vi "5785_IQ_gen_2_x_400MHz_max_transfer_back.vi"() -> ()   [LabVIEW 2021]
uses:
  <instrlib>/_niInstr/Streaming/v1/Common/Stream State.ctl
  <vilib>/Platform/TimedLoop/XDataNode/timing_clust.ctl
  <vilib>/Platform/TimedLoop/XDataNode/nitl_modes.ctl
  <vilib>/Platform/TimedLoop/XDataNode/wakeup.ctl
  <instrlib>/FlexRIO/API/FPGA/v1/Types/Start Trigger IO Resources.ctl
  <instrlib>/_niInstr/DSP/v1/Shared/Public/IQ Data.ctl
  <vilib>/rvi/Emulation/niFpgaSctlEmulationGetInTimedLoop.vi
  <vilib>/rvi/Emulation/niFpgaEmulationReportErrorSimple.vi
  <vilib>/rvi/Emulation/niFpgaGetClockAttributes.vi
  <vilib>/rvi/Emulation/niFpgaCriticalErrorInLSC.vi
  <vilib>/rvi/interface/RandomDataEmulation/nirviRandomDataMultiElementFPGAFIFO.vi
  <instcachedir>/0/nirviRandomDataMultiElementFPGAFIFO_3E9965BA1FAD4E7B8DABA31768A09B1F.lvgen/nirviRandomDataMultiElementFPGAFIFO_3E9965BA1FAD4E7B8DABA31768A09B1F_000.vi
  <vilib>/rvi/interface/RandomDataEmulation/niFpgaRandomDataHandleErrors.vi
  7192f61d-e408-4cca-baff-cb10c33219c0.vi
  <instrlib>/_niInstr/DSP/v1/FPGA/Public/Sub VIs/HB Interpolator/Halfband Interpolator - IQ - 2 SPC - 2x OC.vi
  <instrlib>/_niInstr/DSP/v1/FPGA/Public/Sub VIs/Frequency Shift/Frequency Shift - 4 spc.vi
  <instrlib>/_niInstr/DSP/v1/FPGA/Public/Sub VIs/HB Interpolator/Halfband Interpolator - IQ - 4 SPC - 2x OC.vi
  <instrlib>/_niInstr/DSP/v1/FPGA/Public/Sub VIs/HB Interpolator/Halfband Interpolator - IQ - 8 SPC - 2x OC.vi
  <instrlib>/_niInstr/DSP/v1/FPGA/Public/Sub VIs/Frequency Shift/Frequency Shift - 16 spc.vi
  <instrlib>/_niInstr/DSP/v1/FPGA/Public/Sub VIs/HB Decimator/Halfband Decimator - IQ - 16 spc - 2x oc.vi
  <instrlib>/_niInstr/DSP/v1/FPGA/Public/Sub VIs/HB Decimator/Halfband Decimator - IQ - 8 spc - 2x oc.vi
  <instrlib>/_niInstr/DSP/v1/FPGA/Public/Sub VIs/HB Decimator/Halfband Decimator - IQ - 4 spc - 2x oc.vi
  <instrlib>/_niInstr/DSP/v1/FPGA/Public/Sub VIs/Data Conversion/IQ to U32 - 1 spc - S18.1.vi
  <instrlib>/_niInstr/Basic Elements/v1/FPGA/Private/Count Down U32.vi
  <instcachedir>/0/nirviRandomDataMultiElementFPGAFIFO_3E9965BA1FAD4E7B8DABA31768A09B1F.lvgen/nirviRandomDataMultiElementFPGAFIFO_3E9965BA1FAD4E7B8DABA31768A09B1F_003.vi
  <vilib>/rvi/eio/common/nirviEmuTemplateMethod_errors.vi
  <vilib>/Platform/TimedLoop/XDataNode/XDataNode.xnode
  <vilib>/rvi/DataTransferAndStorage/Container/XNode/niFpgaContainer.xnode
  <vilib>/rvi/interface/RandomDataEmulation/nirviRandomDataFpgaMultiElementTemplate.vi
  <vilib>/eio/EIONode/EIONode.xnode
  <vilib>/Platform/TimedLoop/XDataNode/XDNodeRunTimeDep.lvlib
  <instrlib>/_niInstr/Streaming/v1/FPGA/niInstr Streaming v1 FPGA.lvlib
  <instrlib>/FlexRIO/API/FPGA/v1/FlexRIO API FPGA v1.lvlib
  <instrlib>/FlexRIO/API/FPGA/v1/IO/NI5785/FlexRIO 5785 FPGA v1.lvlib
  <instrlib>/_niInstr/DSP/v1/FPGA/niInstr DSP v1 FPGA.lvlib
  <instrlib>/_niInstr/Basic Elements/v1/FPGA/niInstr Basic Elements v1 FPGA.lvlib
  <instrlib>/_niInstr/DSP/v1/Shared/niInstr DSP v1 Shared.lvlib
  <instrlib>/_niInstr/Streaming/v1/Common/niInstr Streaming v1 Common.lvlib
panel:
  out "Is Rx completed":bool
  out "fifo overflow":bool
  in  "rx count .5":u32
  in  "flexrio.stream.channels enabled 1":u64
  in  "frequency shift Tx":fxp<+/-,48,0>
  in  "frequency shift Rx":fxp<+/-,48,0>
  out "pulse TX status 2":T1
  out "pulse TX status":T1
  in  "reset system clock":bool
  in  "User-defined Start Trigger - AO":bool
  in  "flexrio.trigger.start.cfg 1":u16
  out "IO Socket\\AO Ready For Input":bool
  in  "stream.request state 1":T2
  in  "stream.num samples 1":u64
  out "stream.metadata 1":u64
  out "stream.samples transferred 1":u64
  out "stream.state 1":T2
  out "flexrio.module.io ready 0":bool
  out "flexrio.module.io error 0":i32
  out "flexrio.module.data valid 0":bool
  # "Data Path Configuration"
  # "AI Trigger Configuration"
  # "AI Stream Configuration"
  # "AO Stream Configuration"
  # "Module Status"
  # "AO Buffer Configuration"
  # "User-defined Controls"
  # "AO Trigger Configuration"
  # "5785 KU060"
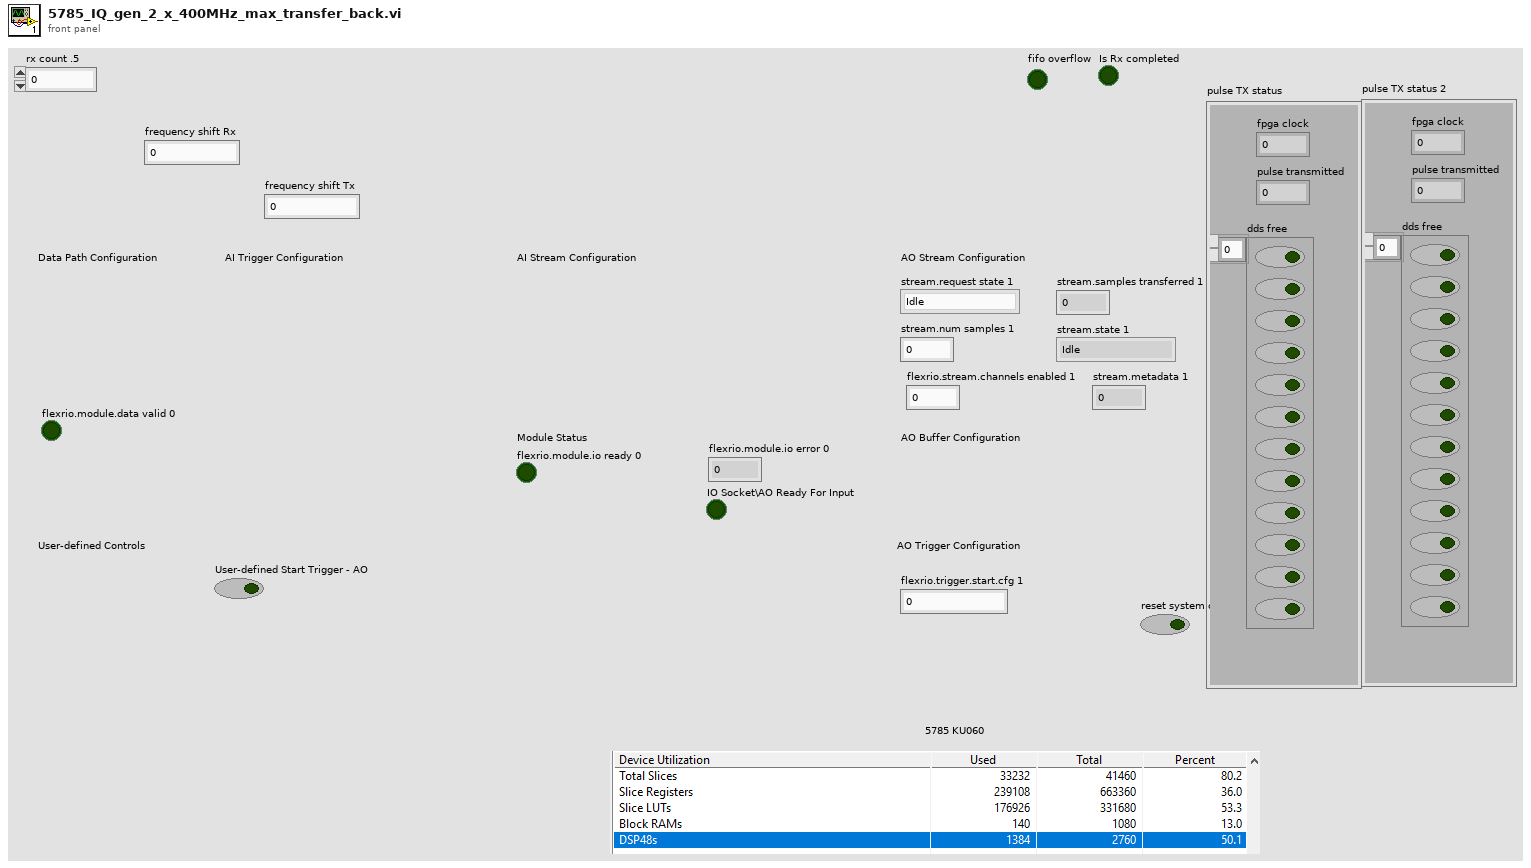
[diagram p1: front panel]
types:
  T1 = cluster{"fpga clock":u64, "pulse transmitted":u32, "dds free":bool[]}
  T2 = typedef "niInstr Streaming v1 Common.lvlib/Stream State.ctl" = enum8{"Idle", "Finite Transfer", "Continuous", "Done", "Error", "Not Ready", "Cancel"}
  T3 = typedef "XDNodeRunTimeDep.lvlib/timing_clust.ctl" = cluster{"Expected End [f-1]":u64, "Actual End [f-1]":u64, "Finished Late? [f-1]":bool, "Expected End [i-1]":u64, "Actual End [i-1]":u64, "Finished Late? [i-1]":bool, "Expected Start [i]":u64, "Actual Start [i]":u64, "Expected Start [f]":u64, "Actual Start [f]":u64, "Source Name":string, "Structure Name":string, "Period":i64, "Deadline":i64, "Offset":i64, "Start":i64, "Priority":i32, "Timeout":i32, "Mode":T4, "Wakeup Reason":T5, "Error":errorcluster, "Source Type":string, "Secondary Source Type":string, "Global End Time":u64, "Global Start Time":u64, "Frame Duration":u64, "Iteration Duration":u64, "Assigned CPU":i32, "I/O Scan Engine Mode":u32}
  T4 = typedef "XDNodeRunTimeDep.lvlib/nitl_modes.ctl" = enum32{"No Change", "Process missed periods, maintain original phase", "Discard missed periods, maintain original phase", "Process missed periods, ignore original phase", "Discard missed periods, ignore original phase"}
  T5 = typedef "XDNodeRunTimeDep.lvlib/wakeup.ctl" = enum32{"Normal", "Aborted", "Asynchronous wakeup", "Timing source error", "Timed loop error", "Timeout"}
  T6 = typedef "FlexRIO API FPGA v1.lvlib/Start Trigger IO Resources.ctl" = cluster{"start trigger":refnum<k21>, "started event":refnum<k21>, "start trigger for export":refnum<k21>, "start trigger for tclk":refnum<k21>}
  T7 = typedef "niInstr DSP v1 Shared.lvlib/IQ Data.ctl" = cluster{"I":fxp<+/-,18,1>, "Q":fxp<+/-,18,1>, "overflow":bool}
  T8 = typedef "FlexRIO API FPGA v1.lvlib/Start Trigger Control.ctl" = cluster{"arm start":bool, "done":bool}
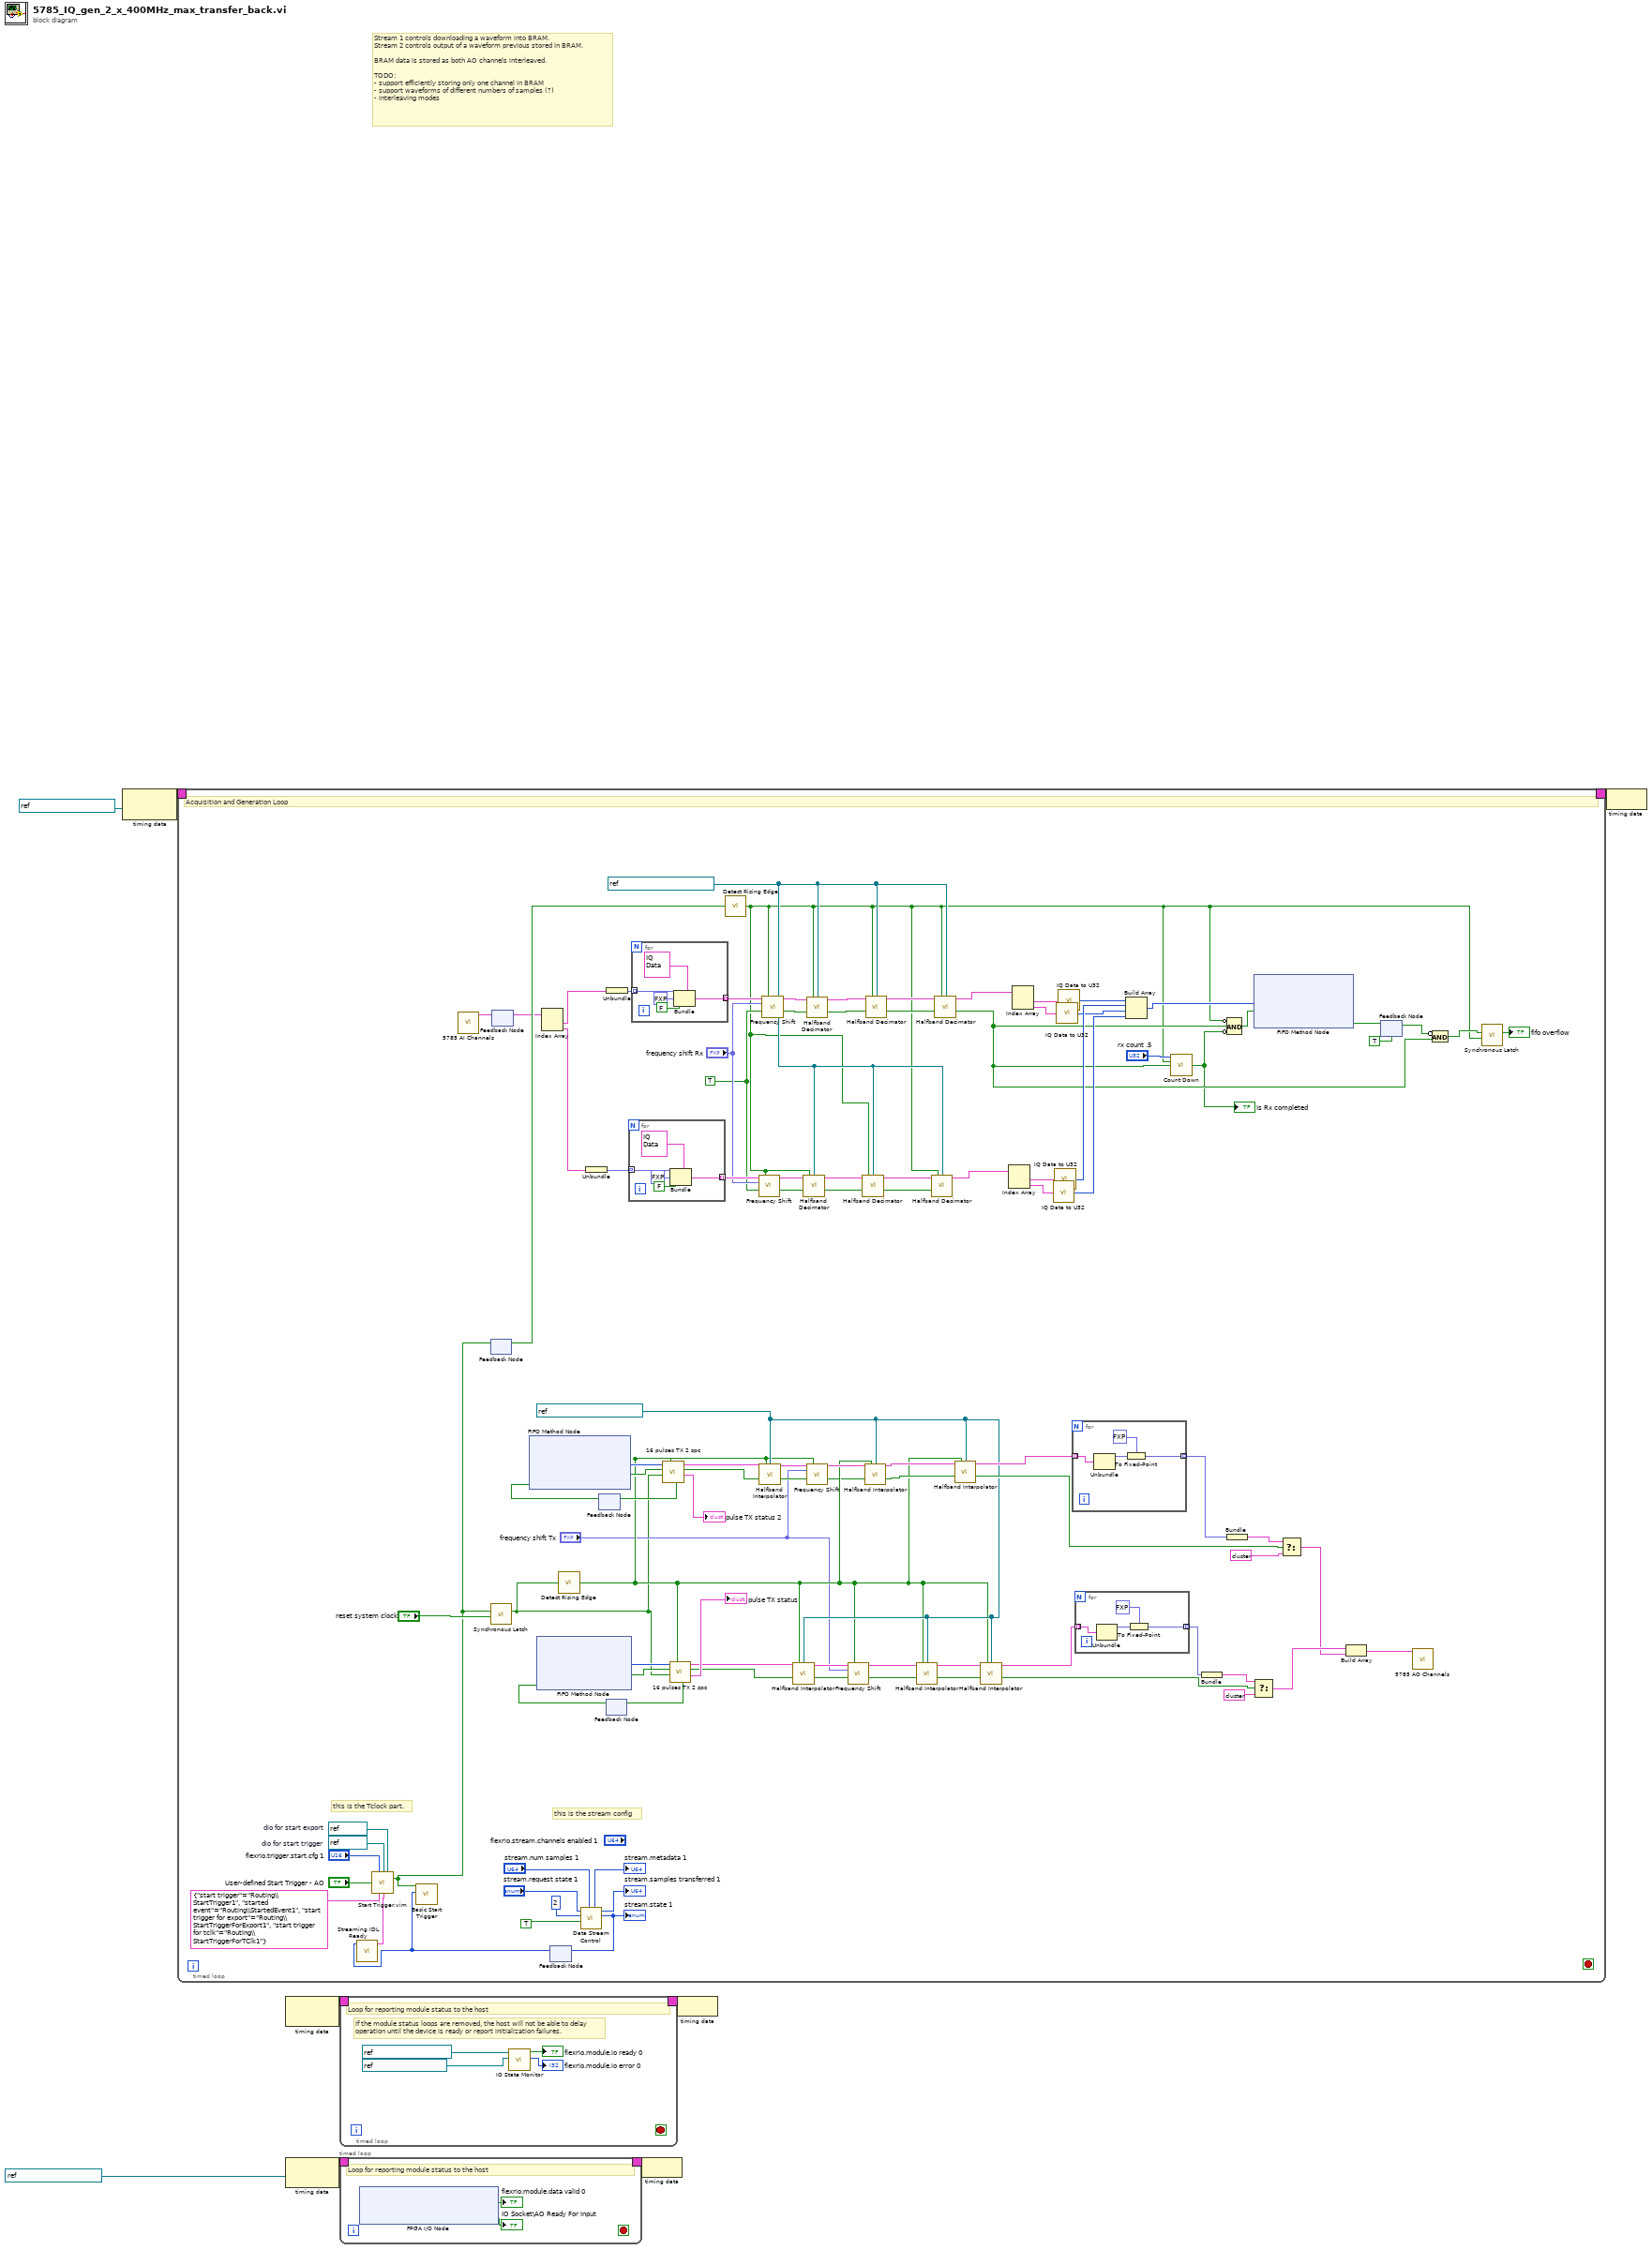
[diagram p0: block diagram]
diagram:
  # "Stream 1 controls downloading a waveform into BRAM.\nStream 2 controls output of a waveform previous stored in BRAM.\n\nBRAM data is stored as both AO channels interleaved.\n\nTODO:\n- support efficiently storing only one channel in BRAM\n- support waveforms of different numbers of samples (?)\n- interleaving modes"
  n1 = node-c288(refnum<k21> "IO Socket\\Data Clock" ("Source Name")) -> (w8:T3)
  n2 = timed-loop {
    timing: w8 -> [_]
    timing-out: [_] -> w7
    stop <- _ stop-if-true
    w22 = TRUE ("input valid")
    w63 = refnum<k21> "IO Socket\\Data Clock 2x" ("clock x 2")
    w52 = refnum<k21> "IO Socket\\Data Clock 2x" ("Source Name")
    w110 = refnum<k21> "DIO 2"  # dio for start trigger
    w109 = refnum<k21> "DIO 3"  # dio for start export
    # "this is the stream config"
    # "this is the Tclock part."
    # "Acquisition and Generation Loop"
    n3 = call <instrlib>:"5785 AI Channels.vi"() -> ("all channels"=w60:cluster{fxp<+/-,12,1>[]}[])  [unwired: 15 in]
    n4 = feedback #1() -> (w61:bool)  [unwired: 1 in]
    n5 = feedback #2() -> (w59:cluster{fxp<+/-,12,1>[]}[])  [unwired: 1 in]
    n6 = feedback-in #2(w60) -> ()
    n7 = Index Array(array=w59) -> (element #1=w83:cluster{fxp<+/-,12,1>[]}, element #2=w62:cluster{fxp<+/-,12,1>[]})  [unwired: 2 in]
    n8 = feedback #3() -> (w10:T2)  [unwired: 1 in]
    n9 = call <instrlib>:"Streaming IDL Ready.vi"("stream.state"=w10) -> ("start trigger control"=w23:T8)  [unwired: 10 in]
    n10 = call "Start Trigger.vim"("flexrio.trigger.start.cfg 0"="flexrio.trigger.start.cfg 1", "dio start"=w110, "dio for start export"=w109, "user-defined start trigger"="User-defined Start Trigger - AO", "trigger io resources"=T6 {"start trigger"="Routing\\StartTrigger1", "started event"="Routing\\StartedEvent1", "start trigger for export"="Routing\\StartTriggerForExport1", "start trigger for tclk"="Routing\\StartTriggerForTClk1"}, "start trigger control"=w23) -> ("conditioned start trigger"=w9:bool)  [unwired: 7 in, 2 out]
    n11 = call <instrlib>:"Basic Start Trigger.vi"("stream.state"=w10, "start trigger"=w9) -> ()  [unwired: 9 in, 1 out]
    n12 = feedback-in #1(w9) -> ()
    n13 = call <instrlib>:"Synchronous Latch.vi"("clear"="reset system clock", "set"=w9) -> ("out"=w35:bool)  [unwired: 9 in]
    n14 = call <instrlib>:"Detect Rising Edge.vi"("signal"=w35) -> ("edge detected"=w38:bool)  [unwired: 14 in]
    n15 = call <instrlib>:"Data Stream Control.vi"("stream.num samples 0"="stream.num samples 1", "data valid"=TRUE, "element count"=u16 2, "stream.request state 0"="stream.request state 1") -> ("stream.state 0"=w11:T2, "stream.samples transferred 0"=→"stream.samples transferred 1":u64, "stream.metadata 0"=→"stream.metadata 1":u64)  [unwired: 3 in, 2 out]
    "stream.state 1" <- w11
    n16 = feedback-in #3(w11) -> ()
    n17 = Unbundle(w62) -> (w67:fxp<+/-,12,1>[])
    n18 = feedback #4() -> (w102:bool)  [unwired: 1 in]
    n19 = xnode ("FIFO Method Node")("Ready for Output"=w102) -> ("Element"=w103:u64[], "Output Valid"=w100:bool)  [unwired: 1 in, 1 out]
    n20 = feedback #5() -> (w105:bool)  [unwired: 1 in]
    n21 = xnode ("FIFO Method Node")("Ready for Output"=w105) -> ("Element"=w104:u64[], "Output Valid"=w97:bool)  [unwired: 1 in, 1 out]
    n22 = Unbundle(w83) -> (w84:fxp<+/-,12,1>[])
    n23 = for {
      tunnel: w67 -> [w124] mode=indexing
      tunnel: [w121] -> w68 mode=indexing
      n24 = Bundle(cluster=T7 {"I"=0.0, "Q"=0.0, "overflow"=FALSE} ("IQ"), "I"=w124, "Q"=fxp<+/-,18,1> 0.0, "overflow"=FALSE) -> (w121:T7)
    }
    n25 = for {
      tunnel: w84 -> [w129] mode=indexing
      tunnel: [w126] -> w82 mode=indexing
      n26 = Bundle(cluster=T7 {"I"=0.0, "Q"=0.0, "overflow"=FALSE} ("IQ"), "I"=w129, "Q"=fxp<+/-,18,1> 0.0, "overflow"=FALSE) -> (w126:T7)
    }
    n27 = call "16 pulses TX 2 spc.vi"("reset system clock"=w38, "IQ_run"=w35, "PDW input Valid"=w100, "array PDW"=w103) -> ("pulse TX status"=→"pulse TX status 2":T1, "output valid"=w42:bool, "IQ out"=w50:T7[], "ready for input"=w101:bool)  [unwired: 4 in]
    n28 = feedback-in #4(w101) -> ()
    n29 = call "16 pulses TX 2 spc.vi"("reset system clock"=w38, "IQ_run"=w35, "PDW input Valid"=w97, "array PDW"=w104) -> ("pulse TX status"=→"pulse TX status":T1, "output valid"=w47:bool, "IQ out"=w48:T7[], "ready for input"=w106:bool)  [unwired: 4 in]
    n30 = feedback-in #5(w106) -> ()
    n31 = call <instrlib>:"Detect Rising Edge.vi"("signal"=w61) -> ("edge detected"=w18:bool)  [unwired: 14 in]
    n32 = call-poly <instrlib>:"Frequency Shift.vi"("data in"=w68, "reset"=w18, "frequency shift"="frequency shift Rx", "input valid"=w22) -> ("data out"=w66:T7[], "output valid"=w70:bool)  [unwired: 8 in, 2 out]
    n33 = call-poly <instrlib>:"Halfband Interpolator.vi"("data in"=w50, "reset"=w38, "clock x 2"=w52, "input valid"=w42) -> ("data out"=w40:T7[], "output valid"=w41:bool)  [unwired: 8 in, 2 out]
    n34 = call-poly <instrlib>:"Frequency Shift.vi"("data in"=w82, "reset"=w18, "frequency shift"="frequency shift Rx", "input valid"=w22) -> ("data out"=w85:T7[], "output valid"=w80:bool)  [unwired: 8 in, 2 out]
    n35 = call-poly <instrlib>:"Halfband Interpolator.vi"("data in"=w48, "reset"=w38, "clock x 2"=w52, "input valid"=w47) -> ("data out"=w46:T7[], "output valid"=w44:bool)  [unwired: 8 in, 2 out]
    n36 = call-poly <instrlib>:"Halfband Decimator.vi"("data in"=w66, "reset"=w18, "clock x 2"=w63, "input valid"=w70) -> ("data out"=w64:T7[], "output valid"=w69:bool)  [unwired: 8 in, 2 out]
    n37 = call-poly <instrlib>:"Halfband Decimator.vi"("data in"=w85, "reset"=w18, "clock x 2"=w63, "input valid"=w80) -> ("data out"=w87:T7[], "output valid"=w81:bool)  [unwired: 8 in, 2 out]
    n38 = call-poly <instrlib>:"Frequency Shift.vi"("data in"=w40, "reset"=w38, "frequency shift"="frequency shift Tx", "input valid"=w41) -> ("data out"=w39:T7[], "output valid"=w36:bool)  [unwired: 8 in, 2 out]
    n39 = call-poly <instrlib>:"Frequency Shift.vi"("data in"=w46, "reset"=w38, "frequency shift"="frequency shift Tx", "input valid"=w44) -> ("data out"=w45:T7[], "output valid"=w43:bool)  [unwired: 8 in, 2 out]
    n40 = call-poly <instrlib>:"Halfband Decimator.vi"("data in"=w64, "reset"=w18, "clock x 2"=w63, "input valid"=w69) -> ("data out"=w65:T7[], "output valid"=w71:bool)  [unwired: 8 in, 2 out]
    n41 = call-poly <instrlib>:"Halfband Interpolator.vi"("data in"=w39, "reset"=w38, "clock x 2"=w52, "input valid"=w36) -> ("data out"=w57:T7[], "output valid"=w51:bool)  [unwired: 8 in, 2 out]
    n42 = call-poly <instrlib>:"Halfband Decimator.vi"("data in"=w87, "reset"=w18, "clock x 2"=w63, "input valid"=w81) -> ("data out"=w86:T7[], "output valid"=w79:bool)  [unwired: 8 in, 2 out]
    n43 = call-poly <instrlib>:"Halfband Interpolator.vi"("data in"=w45, "reset"=w38, "clock x 2"=w52, "input valid"=w43) -> ("data out"=w56:T7[], "output valid"=w55:bool)  [unwired: 8 in, 2 out]
    n44 = call-poly <instrlib>:"Halfband Decimator.vi"("data in"=w65, "reset"=w18, "clock x 2"=w63, "input valid"=w71) -> ("data out"=w72:T7[])  [unwired: 8 in, 3 out]
    n45 = call-poly <instrlib>:"Halfband Decimator.vi"("data in"=w86, "reset"=w18, "clock x 2"=w63, "input valid"=w79) -> ("data out"=w78:T7[], "output valid"=w21:bool)  [unwired: 8 in, 2 out]
    n46 = call-poly <instrlib>:"Halfband Interpolator.vi"("data in"=w57, "reset"=w38, "clock x 2"=w52, "input valid"=w51) -> ("data out"=w98:T7[], "output valid"=w99:bool)  [unwired: 8 in, 2 out]
    n47 = call-poly <instrlib>:"Halfband Interpolator.vi"("data in"=w56, "reset"=w38, "clock x 2"=w52, "input valid"=w55) -> ("data out"=w53:T7[], "output valid"=w54:bool)  [unwired: 8 in, 2 out]
    n48 = Index Array(array=w72) -> (element #1=w73:T7, element #2=w74:T7)  [unwired: 2 in]
    n49 = Index Array(array=w78) -> (element #1=w77:T7, element #2=w76:T7)  [unwired: 2 in]
    n50 = call-poly <instrlib>:"IQ Data to U32.vi"("IQ data"=w74) -> ("U32 data"=w27:u32)  [unwired: 13 in, 1 out]
    n51 = call-poly <instrlib>:"IQ Data to U32.vi"("IQ data"=w73) -> ("U32 data"=w26:u32)  [unwired: 13 in, 1 out]
    n52 = call-poly <instrlib>:"IQ Data to U32.vi"("IQ data"=w76) -> ("U32 data"=w25:u32)  [unwired: 13 in, 1 out]
    n53 = call-poly <instrlib>:"IQ Data to U32.vi"("IQ data"=w77) -> ("U32 data"=w75:u32)  [unwired: 13 in, 1 out]
    n54 = for {
      tunnel: w98 -> [w116] mode=indexing
      tunnel: [w113] -> w95 mode=indexing
      n55 = Unbundle(w116) -> ("I"=w115:fxp<+/-,18,1>)  [unwired: 2 out]
      n56 = To Fixed-Point(fixed-point type=fxp<+/-,12,1> 0.0 ("element"), number=w115) -> (fixed-point=w113:fxp<+/-,12,1>)
    }
    n57 = for {
      tunnel: w53 -> [w120] mode=indexing
      tunnel: [w117] -> w96 mode=indexing
      n58 = Unbundle(w120) -> ("I"=w119:fxp<+/-,18,1>)  [unwired: 2 out]
      n59 = To Fixed-Point(fixed-point type=fxp<+/-,12,1> 0.0 ("element"), number=w119) -> (fixed-point=w117:fxp<+/-,12,1>)
    }
    n60 = Build Array(w75, w26, w25, w27) -> (w28:u32[])
    n61 = call-poly <instrlib>:"Count Down.vi"("count in"="rx count .5", "load"=w18, "decrement"=w21) -> ("terminal count"=w19:bool)  [unwired: 11 in, 1 out]
    "Is Rx completed" <- w19
    n62 = Bundle(w96) -> (w94:cluster{fxp<+/-,12,1>[]})  [unwired: 1 in]
    n63 = Compound Arithmetic op=AND(invert w18, w21, invert w19) -> (w20:bool)
    n64 = Bundle(w95) -> (w90:cluster{fxp<+/-,12,1>[]})  [unwired: 1 in]
    n65 = Select(t=w94, s=w54, f=cluster{fxp<+/-,12,1>[]} {[0.0, 0.0, 0.0, 0.0, 0.0, 0.0, 0.0, 0.0, 0.0, 0.0, 0.0, 0.0, 0.0, 0.0, 0.0, 0.0]}) -> (s? t:f=w93:cluster{fxp<+/-,12,1>[]})
    n66 = xnode ("FIFO Method Node")("Element"=w28, "Input Valid"=w20) -> ("Ready for Input"=w29:bool)  [unwired: 1 in, 1 out]
    n67 = Select(t=w90, s=w99, f=cluster{fxp<+/-,12,1>[]} {[0.0, 0.0, 0.0, 0.0, 0.0, 0.0, 0.0, 0.0, 0.0, 0.0, 0.0, 0.0, 0.0, 0.0, 0.0, 0.0]}) -> (s? t:f=w89:cluster{fxp<+/-,12,1>[]})
    n68 = Build Array(w93, w89) -> (w112:cluster{fxp<+/-,12,1>[]}[])
    n69 = feedback-in #6(w29) -> ()
    n70 = feedback #6(TRUE ("Ready for Input")) -> (w32:bool)
    n71 = call <instrlib>:"5785 AO Channels.vi"("all channels"=w112) -> ()  [unwired: 15 in]
    n72 = Compound Arithmetic op=AND(invert w32, w21) -> (w31:bool)
    n73 = call <instrlib>:"Synchronous Latch.vi"("clear"=w18, "set"=w31) -> ("out"=→"fifo overflow":bool)  [unwired: 9 in]
  }
  n74 = node-c288() -> (w5:T3)  [unwired: 1 in]
  n75 = node-c288(refnum<k21> "IO Socket\\Data Clock" ("Source Name")) -> (w3:T3)
  n76 = timed-loop {
    timing: w5 -> [_]
    timing-out: [_] -> w4
    stop <- _ stop-if-true
    # "If the module status loops are removed, the host will not be able to delay operation until the device is ready or report initialization failures."
    # "Loop for reporting module status to the host"
    n77 = call <instrlib>:"IO State Monitor.vi"("io error resource"=refnum<k21> "IO Socket\\IO Error" ("FPGA I/O In"), "io ready resource"=refnum<k21> "IO Socket\\IO Ready" ("FPGA I/O In")) -> ("flexrio.module.io error 0"=→"flexrio.module.io error 0":i32, "flexrio.module.io ready 0"=→"flexrio.module.io ready 0":bool)  [unwired: 8 in]
  }
  n78 = timed-loop {
    timing: w3 -> [_]
    timing-out: [_] -> w2
    stop <- _ stop-if-true
    # "Loop for reporting module status to the host"
    n79 = xnode "FPGA I/O Node"() -> ("IO Socket\\AI Data Valid"=→"flexrio.module.data valid 0":bool, "IO Socket\\AO Ready For Input"=→"IO Socket\\AO Ready For Input":bool)  [unwired: 2 in, 2 out]
  }
  n80 = node-c288(w2) -> ()
  n81 = node-c288(w4) -> ()
  n82 = node-c288(w7) -> ()
